vi "Get Version Number.vi"(8 "error in (no error)":errorcluster, 11 "DB-Interface in":refnum<class "DB-Interface.lvclass">) -> (0 "error out":errorcluster, 2 "Version Number":string, 3 "DB-Interface out":refnum<class "DB-Interface.lvclass">)   [LabVIEW 2020, in "hse-db.lvlib" / "DB-Interface.lvclass"]
doc: "____\nHAMPEL SOFTWARE ENGINEERING v1.4.0 (2023-12-19 09:52)"
uses:
  DB-Interface.lvclass
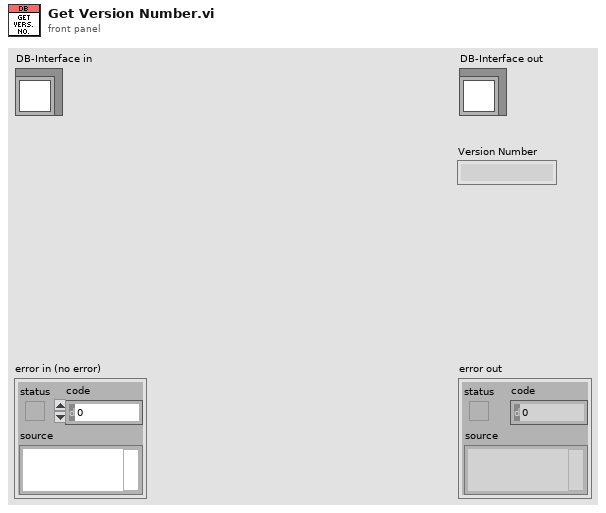
[diagram p1: front panel]
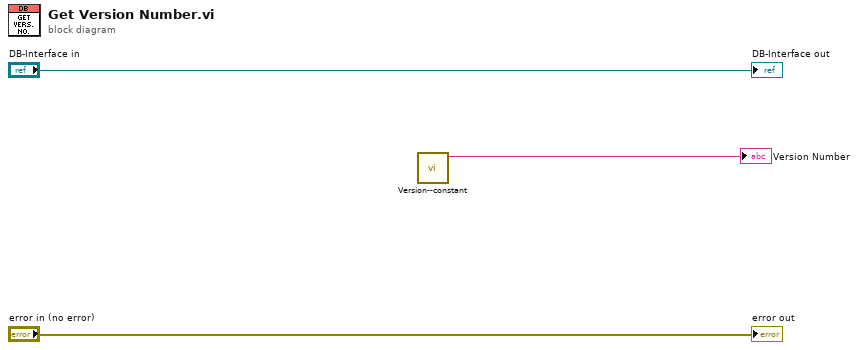
[diagram p0: block diagram]
diagram:
  n1 = call "Version--constant.vi"() -> ("Version Number"=→"Version Number":string)  [unwired: 11 in]
  "error out" <- "error in (no error)"
  "DB-Interface out" <- "DB-Interface in"
